vi "Global_ACT_Data Out.vi"() -> ()   [LabVIEW 2023, in "2024 AdvSwerve_ACT.lvlib"]
uses:
  2024 AdvSwerve_ACT.lvlib
  Cluster_HW Output Values.ctl
  Cluster_System Output Data.ctl
  ENUM_ACT_State.ctl
  Shared Code/TypeDefs/Dial_Compase heading unit circle CCW positive.ctl
  Shared Code/TypeDefs/Level_Velocity plus-minus 1.ctl
  Shared Code/TypeDefs/Cluster_Module Velocity-Direction-Rotations.ctl
  Shared Code/TypeDefs/Cluster_Swerve 4 Steer and Velocity.ctl
panel:
  out "ACT_Template_STATE":T1
  in  "ACT_Template_System Output":T2
  out "ACT_Template_HW Output":T3 {"Swerve Read"."Back Right"."Angle" scale format="%.3f"; "Swerve Read"."Back Right"."Velocity" scale=-1.0..1.0 scale format="%.1f"; "Swerve Read"."Back Left"."Angle" scale format="%.3f"; "Swerve Read"."Back Left"."Velocity" scale=-1.0..1.0 scale format="%.1f"; "Swerve Read"."Front Left"."Angle" scale format="%.3f"; "Swerve Read"."Front Left"."Velocity" scale=-1.0..1.0 scale format="%.1f"; "Swerve Read"."Front Right"."Angle" scale format="%.3f"; "Swerve Read"."Front Right"."Velocity" scale=-1.0..1.0 scale format="%.1f"; "Pigeon Heading" scale format="%.3f"}
  in  "ACT_Template_CycleTime(S)":dbl
  # "The Names of the Data items in the Global Variable MUST describe who the Single Writer is\nFor Actuator Globals the the naming convention is\n   \nACT_Lib Name_Data Name\n\nExamples:\nACT_Drive_X axis\nACT_Hopper_AgitatorSpeed"
  # "\"Front\" of Robot"
  # "Index 1"
  # "Index 0"
  # "Index 3"
  # "Index 2"
  # "Right Hand Rule"
  # "X"
  # "+CCW"
  # "Y"
  # "(0,0)"
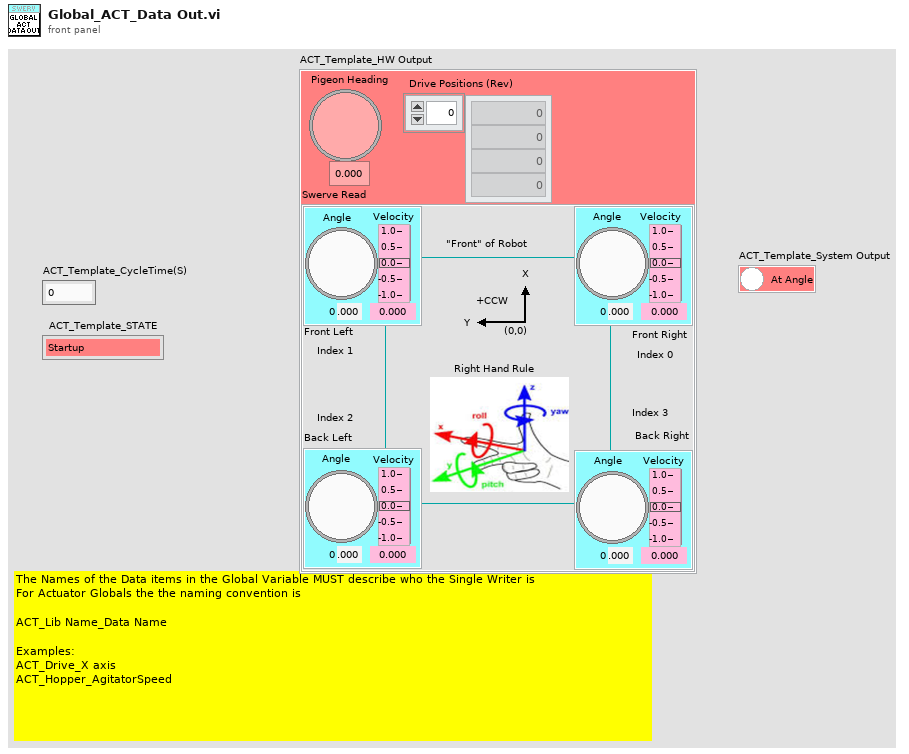
[diagram p1: front panel]
types:
  T1 = typedef "2024 AdvSwerve_ACT.lvlib/ENUM_ACT_State.ctl" = enum16{"Startup", "Configuring", "Stopping", "Moving Mode 1", "Moving Mode 2", "Shutdown", "Initializing HW"}
  T2 = typedef "2024 AdvSwerve_ACT.lvlib/Cluster_System Output Data.ctl" = cluster{"At Angle":bool}
  T3 = typedef "2024 AdvSwerve_ACT.lvlib/Cluster_HW Output Values.ctl" = cluster{"Pigeon Heading":T4, "Swerve Read":T5, "Drive Positions (Rev)":dbl[]}
  T4 = typedef "Dial_Compase heading unit circle CCW positive.ctl" = dbl
  T5 = typedef "Cluster_Swerve 4 Steer and Velocity.ctl" = cluster{"Front Right":T6, "Front Left":T6, "Back Left":T6, "Back Right":T6}
  T6 = typedef "Cluster_Module Velocity-Direction-Rotations.ctl" = cluster{"Velocity":T7, "Angle":T4, "Rotations Count":dbl}
  T7 = typedef "Level_Velocity plus-minus 1.ctl" = dbl
diagram:
